vi "TipoBarrido.vi"(2 "Tipo":enum16{"Simple", "Zig-Zag", "Retorno"}(ring), 3 "Par":bool, 4 "Array Y":dbl[](array[numeric])) -> (0 "Arr Pos":i32[](array[numeric]))   [LabVIEW 2018]
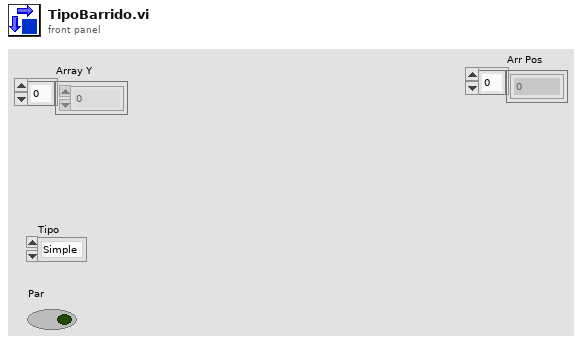
[diagram p1: front panel]
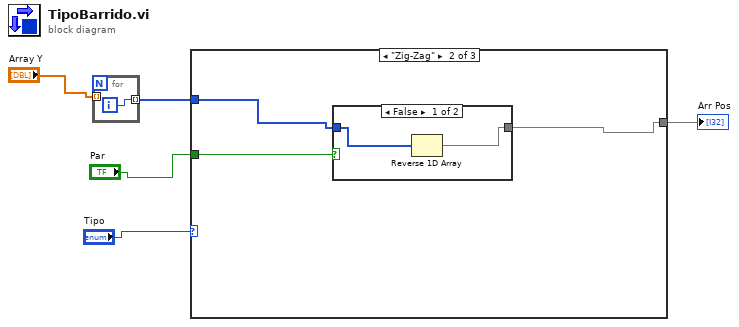
[diagram p0: block diagram]
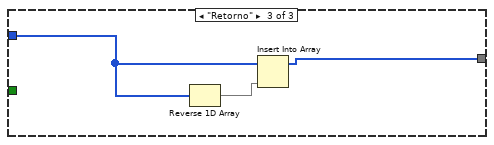
[diagram p4: hidden frame]
diagram:
  n1 = for {
    tunnel: "Array Y" -> [_] mode=indexing
    tunnel: [w6] -> w2 mode=indexing
    i -> [w6]
  }
  n2 = case shown="\"Zig-Zag\"" "Tipo" {
    tunnel: [w7 w8 w16] -> w4
    tunnel: w2 -> [w7 w9 w15]
    tunnel: "Par" -> [_ w10 _]
    frame "Simple", Default {
    }
    frame "Zig-Zag" {
      n3 = case shown="False" w10 {
        tunnel: w9 -> [w12 w13]
        tunnel: [w11 w13] -> w8
        frame False {
          n4 = Reverse 1D Array(array=w12) -> (reversed array=w11:i32[])
        }
        frame True {
        }
      }
    }
    frame "Retorno" {
      n5 = Reverse 1D Array(array=w15) -> (reversed array=w14:i32[])
      n6 = Insert Into Array(array=w15, new element=w14) -> (w16:i32[])  [unwired: 1 in]
    }
  }
  "Arr Pos" <- w4
